vi "New Actor Message Transport.vi"(7 "Return Priority (Normal)":T1=enum."Normal", 9 "Datum Name":string, 10 "Desired Notification Msg (Type)":refnum<class "Notification Msg.lvclass">, 11 "Message Enqueuer in":refnum<class "Message Enqueuer.lvclass">) -> (0 "error out":errorcluster, 3 "ActorMessage out":refnum<class "ActorMessage.lvclass">)   [LabVIEW 2015, in "Transport.lvlib" / "ActorMessage.lvclass"]
doc: "<License>\nCopyright © 2017 Composed Systems, LLC | All rights reserved\nwww.composed.io\n\nAuthor: Ethan Stern <ethan.stern@composed.io>\n\nThis software is provided \"AS IS\" WITHOUT WARRANTIES, either express or implied, AND IS FOR EDUCATIONAL PURPOSES ONLY.\n</License>"
uses:
  ActorMessage.lvclass
  Transport Messages/Notification Msg/Notification Msg.lvclass
  <vilib>/ActorFramework/Message Enqueuer/Message Priority.ctl
  <vilib>/ActorFramework/Message Enqueuer/Message Enqueuer.lvclass
  ActorMessage.lvclass/ActorMessage.ctl
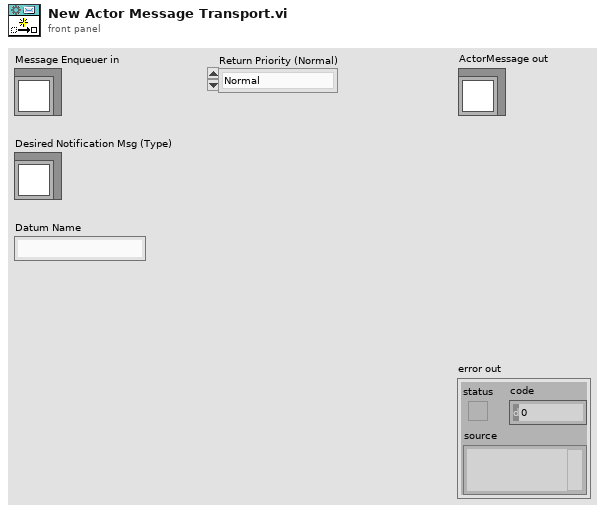
[diagram p1: front panel]
types:
  T1 = typedef "Actor Framework.lvlib/Message Enqueuer.lvclass/Message Priority.ctl" = enum16{"Low", "Normal", "High"}
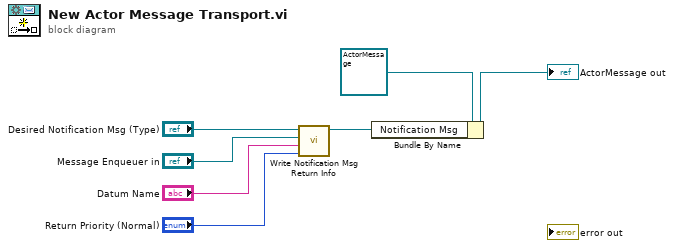
[diagram p0: block diagram]
diagram:
  n1 = call "Write Notification Msg Return Info.vi"("Return Priority (Normal)"="Return Priority (Normal)", "Datum Name"="Datum Name", "Message Enqueuer in"="Message Enqueuer in", "Notification Msg"="Desired Notification Msg (Type)") -> ("Notification Msg Out"=w4:refnum<class "Notification Msg.lvclass">)  [unwired: 7 in]
  n2 = Bundle By Name(cluster=refnum<class "ActorMessage.lvclass"> refnum ("ActorMessage in"), "Notification Msg"=w4) -> (→"ActorMessage out":refnum<class "ActorMessage.lvclass">)
